vi "Normalizer.vi"(0 "Acc":u64[][](array[numeric]), 1 "m":dbl, 4 "p":dbl, 5 "Tamaño Sn":i32[](array[numeric]), 6 "Analysis 2":u16(ring) items=["Auto correlation A", "Auto correlation B", "Cross correlation AxB", "Cross correlation BxA"], 7 "AvgA":dbl, 9 "Time":dbl[](array[numeric]), 10 "DataA":sgl[](array[numeric]), 11 "AvgB":dbl, 12 "DataB":sgl[](array[numeric])) -> (13 "bA_B":dbl, 14 "g(k)_2":dbl[][](array[numeric]), 15 "bA":dbl, 16 "s(k)_n":dbl[][](array[numeric]), 17 "bB":dbl, 18 "s(k)":dbl[][](array[numeric]), 19 "g(k)":dbl[][](array[numeric]))   [LabVIEW 2015]
uses:
  <vilib>/Analysis/Matrix/Numeric/Conversions/Matrix To Array - RM.vi
  <vilib>/Analysis/Matrix/NI_Matrix.lvlib
panel:
  out "X2Tau":dbl[][](array[numeric])
  out "X2i":dbl[][](array[numeric])
  out "element":i32
  out "size(s)":i32[](array[numeric])
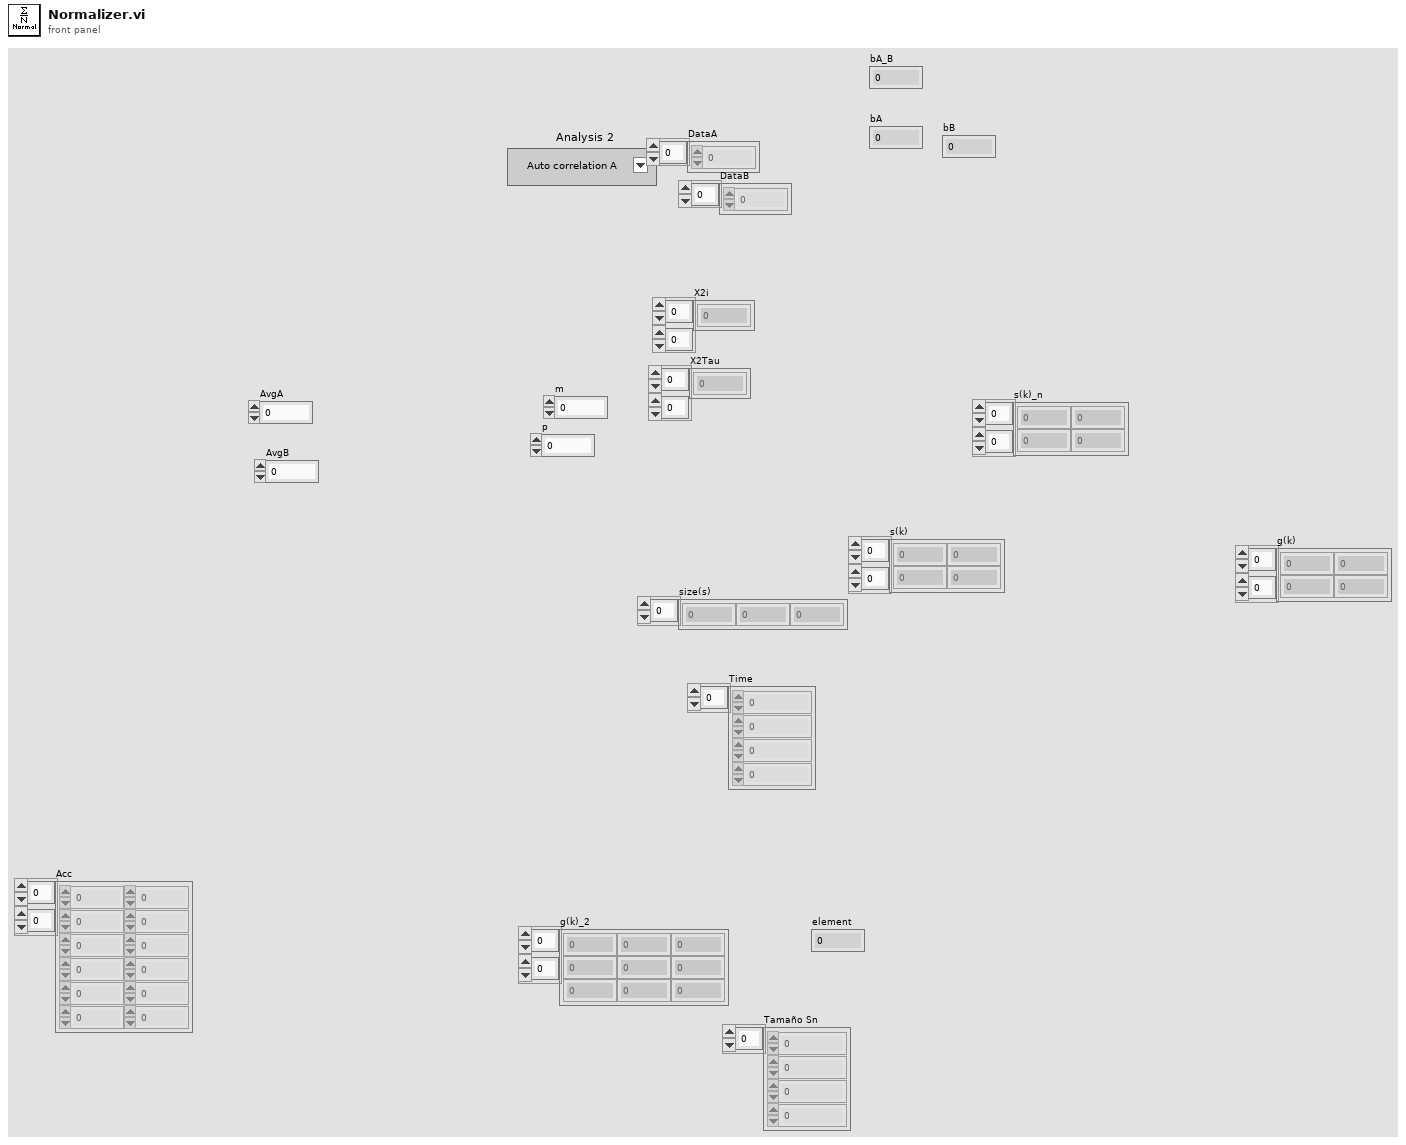
[diagram p1: front panel]
types:
  T1 = typedef "NI_Matrix.lvlib/RealMatrix.ctl" = dbl[][]
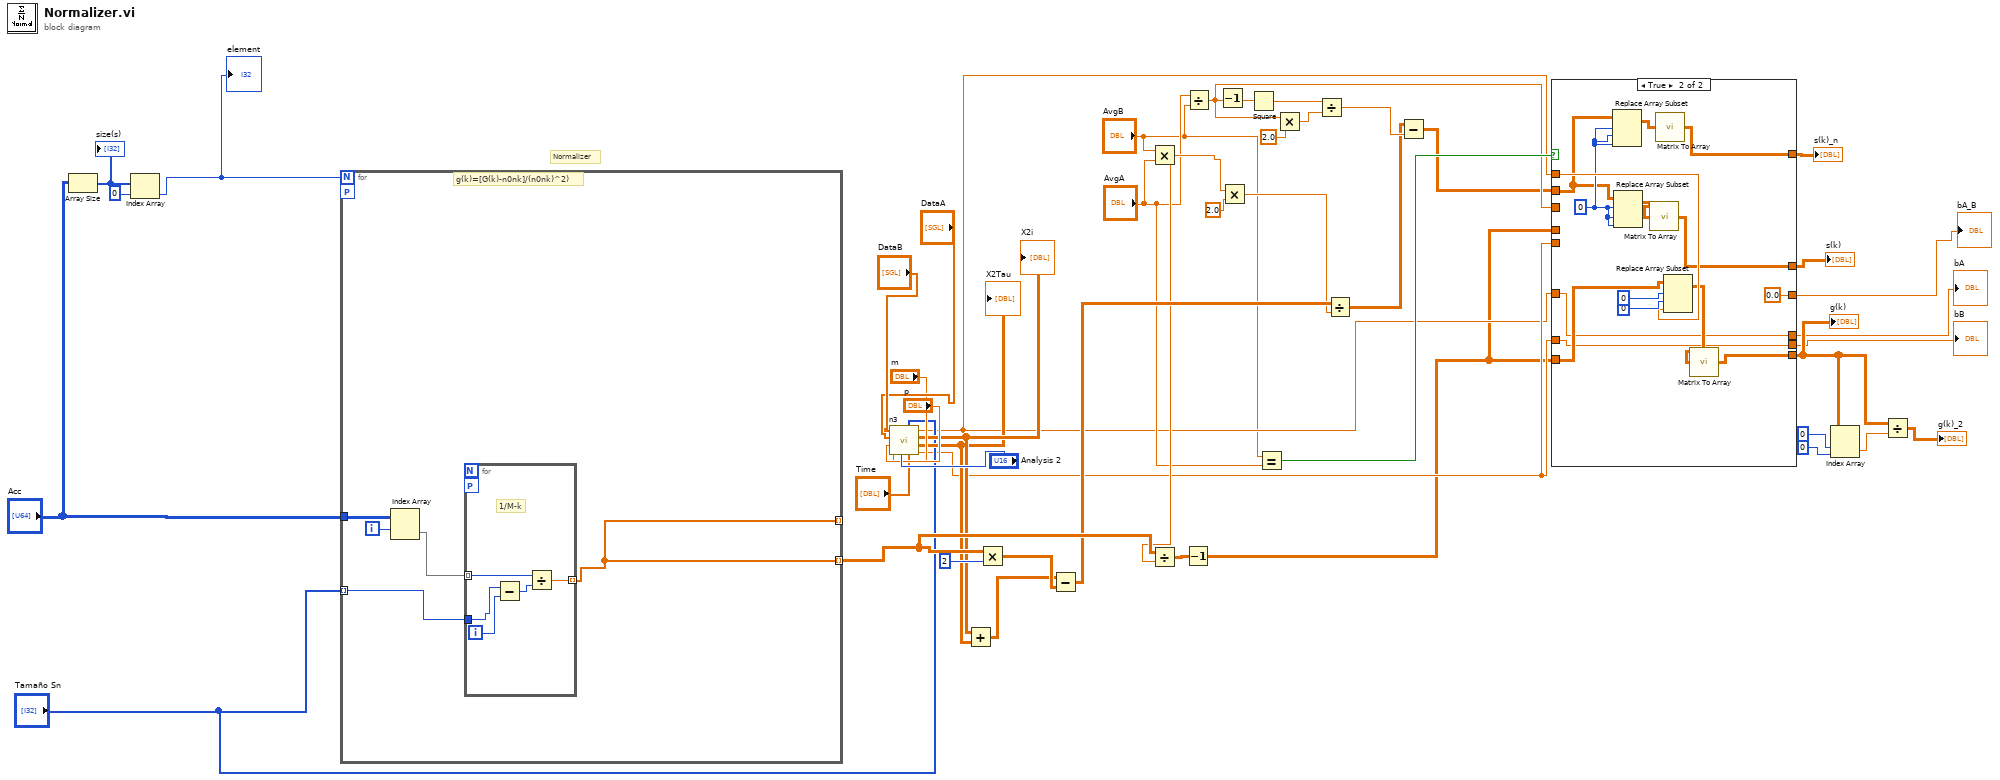
[diagram p0: block diagram]
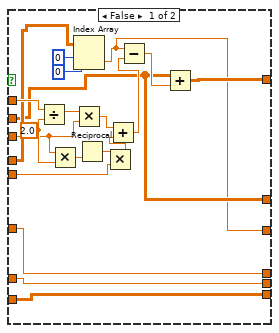
[diagram p2: hidden frame]
diagram:
  # "Normalizer"
  n1 = Array Size(array="Acc") -> (size(s)=w45:i32[])
  "size(s)" <- w45
  n2 = Index Array(array=w45, index=0) -> (element=w21:i32)
  "element" <- w21
  n3 = for {
    N: w21 -> [_]
    tunnel: "Acc" -> [w49]
    tunnel: "Tamaño Sn" -> [w51] mode=indexing
    tunnel: [w47] -> w38 mode=indexing
    tunnel: [w47] -> _ mode=indexing
    workers-P: _ -> [_]
    i -> [w48]
    # "g(k)=[G(k)-n0nk]/(n0nk)^2)"
    n4 = Index Array(array=w49, index (row)=w48) -> (element=w50:u64[])  [unwired: 1 in]
    n5 = for {
      tunnel: [w56] -> w47 mode=indexing
      tunnel: w50 -> [w55] mode=indexing
      tunnel: w51 -> [w53]
      workers-P: _ -> [_]
      i -> [w52]
      # "1/M-k"
      n6 = Subtract(x=w53, y=w52) -> (x-y=w54:i32)
      n7 = Divide(x=w55, y=w54) -> (x/y=w56:dbl)
    }
  }
  n8 = call "n3.vi"("Time"="Time", "Tamaño Sn"="Tamaño Sn", "Analysis"="Analysis 2", "m"="m", "P"="p", "Segmentation A"="DataA", "Segmentation B"="DataB") -> ("bB"=w8:dbl, "X2_tau"=w30:dbl[][], "X2_i"=w31:dbl[][], "bA"=w4:dbl)  [unwired: 1 in]
  "X2i" <- w31
  "X2Tau" <- w30
  n9 = Add(x=w31, y=w30) -> (x+y=w41:dbl[][])
  n10 = Multiply(x=w38, y=2 ("index")) -> (x*y=w42:dbl[][])
  n11 = Subtract(x=w41, y=w42) -> (x-y=w37:dbl[][])
  n12 = Multiply(x="AvgB", y="AvgA") -> (x*y=w17:dbl)
  n13 = Divide(x=w38, y=w17) -> (x/y=w40:dbl[][])
  n14 = Decrement(x=w40) -> (x-1=w1:dbl[][])
  n15 = Divide(x="AvgA", y="AvgB") -> (x/y=w18:dbl)
  n16 = Decrement(x=w18) -> (x-1=w26:dbl)
  n17 = Multiply(x=w17, y=2.0) -> (x*y=w27:dbl)
  n18 = Square(x=w26) -> (x^2=w25:dbl)
  n19 = Equal?(x="AvgB", y="AvgA") -> (x = y?=w20:bool)
  n20 = Multiply(x=w18, y=2.0) -> (x*y=w23:dbl)
  n21 = Divide(x=w25, y=w23) -> (x/y=w22:dbl)
  n22 = Divide(x=w37, y=w27) -> (x/y=w9:dbl[][])
  n23 = Subtract(x=w9, y=w22) -> (x-y=w10:dbl[][])
  n24 = case shown="True" w20 {
    tunnel: w10 -> [w60 w77]
    tunnel: [w63 w81] -> w19
    tunnel: w4 -> [w74 w88]
    tunnel: w18 -> [w71 _]
    tunnel: w8 -> [w68 _]
    tunnel: w1 -> [w62 w91]
    tunnel: [w62 w86] -> w14
    tunnel: w1 -> [w61 _]
    tunnel: [w60 w84] -> w2
    tunnel: w4 -> [w58 w80]
    tunnel: w8 -> [w57 w79]
    tunnel: [w59 0.0] -> w7
    tunnel: [w58 w80] -> w6
    tunnel: [w57 w79] -> w5
    frame False {
      w72 = 2.0 ("y")
      n25 = Divide(x=w74, y=w72) -> (x/y=w73:dbl)
      n26 = Multiply(x=w71, y=w72) -> (x*y=w70:dbl)
      n27 = Index Array(array=w61, index (row)=0, index (col)=0) -> (element=w59:dbl)
      n28 = Multiply(x=w73, y=w71) -> (x*y=w66:dbl)
      n29 = Reciprocal(x=w70) -> (1/x=w69:dbl)
      n30 = Multiply(x=w69, y=w68) -> (x*y=w67:dbl)
      n31 = Add(x=w66, y=w67) -> (x+y=w65:dbl)
      n32 = Subtract(x=w59, y=w65) -> (x-y=w64:dbl)
      n33 = Add(x=w60, y=w64) -> (x+y=w63:dbl[][])
    }
    frame True {
      w82 = 0 ("index (row)")
      n34 = Replace Array Subset(array=w77, new element=w82, index (row)=w82, index (col)=w82) -> (w83:T1)
      n35 = Replace Array Subset(array=w77, new element=w82, index (row)=w82, index (col)=w82) -> (w85:T1)
      n36 = call-poly <vilib>:"Matrix To Array.vi"("Real Matrix"=w85) -> ("Real 2D Array"=w84:dbl[][])
      n37 = call-poly <vilib>:"Matrix To Array.vi"("Real Matrix"=w83) -> ("Real 2D Array"=w81:dbl[][])
      n38 = Replace Array Subset(array=w91, new element=w88, index (row)=0, index (col)=0 ("disabled index (col)")) -> (w87:T1)
      n39 = call-poly <vilib>:"Matrix To Array.vi"("Real Matrix"=w87) -> ("Real 2D Array"=w86:dbl[][])
    }
  }
  "s(k)" <- w2
  "s(k)_n" <- w19
  "g(k)" <- w14
  "bA" <- w6
  "bB" <- w5
  "bA_B" <- w7
  n40 = Index Array(array=w14, index (row)=0, index (col)=0) -> (element=w11:dbl)
  n41 = Divide(x=w14, y=w11) -> (x/y=→"g(k)_2":dbl[][])
